vi "Load_Traverse_Configurations.vi"(11 "Traverse Name":string) -> (3 "Error String":string)   [LabVIEW 2022 SP3]
uses:
  Anemometry/Anemometry Sub Vis/Globals/Constants_global.vi
  DriveConfigGlobal.vi
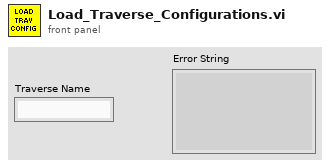
[diagram p1: front panel]
types:
  T1 = cluster{"Channel Name":string, "Vel. Default":sgl, "Acc. Default":sgl, "Vel. Max":sgl, "Vel. Min":sgl, "Acc. Max":sgl, "Acc. Min":sgl, "Pulses/unit":sgl, "Address":u8, "Pulse Offset":i32, "Pos Tolerance":sgl, "Pulses/rev":sgl, "Backlash/Eng units":sgl, "Current Pos":sgl, "Ch Status":enum16{"Active", "Offline", "Simulate"}, "Port Name":string, "Axis Transform mode":string, "Metadata Ch Name":string, "Type":string, "De Power Motor":enum16{"TRUE", "FALSE"}, "ConfigString":string}[]
  T2 = enum16{"Load setup from excel file", "Save setup to excel file"}
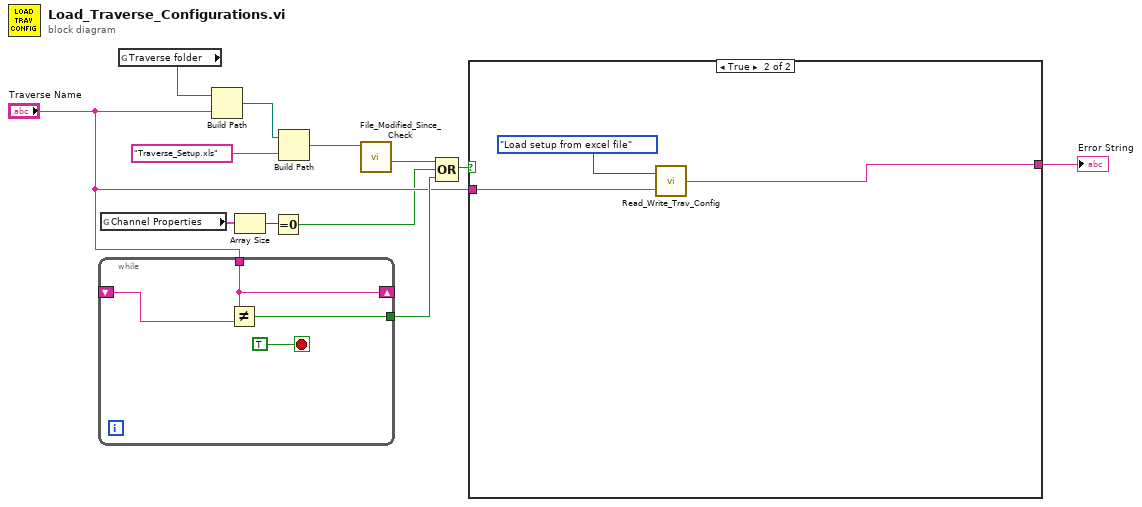
[diagram p0: block diagram]
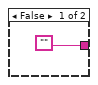
[diagram p2: hidden frame]
diagram:
  n1 = while {
    shift-right: [w14] -> _
    shift-left: _ -> [w15]
    tunnel: "Traverse Name" -> [w14]
    tunnel: [w13] -> w12
    stop <- TRUE stop-if-true
    n2 = Not Equal?(x=w14, y=w15) -> (x != y?=w13:bool)
  }
  n3 = global read "DriveConfigGlobal.vi" "Channel Properties"() -> (w4:T1)
  n4 = global read "Constants_global.vi" "Traverse folder"() -> (w9:path)
  n5 = Build Path(base path=w9, name or relative path="Traverse Name") -> (appended path=w10:path)
  n6 = Array Size(array=w4) -> (size(s)=w5:i32)
  n7 = Equal To 0?(x=w5) -> (x = 0?=w6:bool)
  n8 = Build Path(base path=w10, name or relative path="Traverse_Setup.xls" ("Substring")) -> (appended path=w2:path)
  n9 = call "File_Modified_Since_Check.vi"("File Path"=w2) -> ("modifiedSinceRead"=w1:bool)  [unwired: 7 in, 1 out]
  n10 = Compound Arithmetic op=OR(w1, w6, w12) -> (w7:bool)
  n11 = case shown="True" w7 {
    tunnel: "Traverse Name" -> [_ w19]
    tunnel: ["" w18] -> w3
    frame False {
    }
    frame True {
      n12 = call "Read_Write_Trav_Config.vi"("Traverse Name"=w19, "Mode"=T2."Load setup from excel file") -> ("Error String"=w18:string)
    }
  }
  "Error String" <- w3
